vi "Launcher.vi"   [LabVIEW 2019]
uses:
  EmulatorActor/EmulatorActor/EmulatorActor.lvclass
  C:/Program Files (x86)/National Instruments/LabVIEW 2019/vi.lib/ActorFramework/Actor/Actor.lvclass
  <vilib>/ActorFramework/Actor/Actor.lvclass
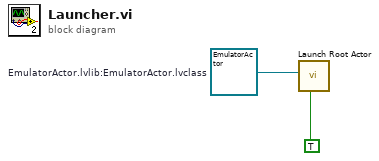
[diagram p0: block diagram]
diagram:
  w2 = refnum<class "EmulatorActor.lvclass"> refnum  # EmulatorActor.lvlib:EmulatorActor.lvclass
  n1 = call <vilib>:"Launch Root Actor.vi"("Open Actor Core front panel? (F)"=TRUE, "Actor"=w2) -> ()  [unwired: 8 in, 2 out]
